vi "USRP SFP.vi"(0 "sfp 0.resources":T2, 5 "sfp 1.resources":T1) -> ()   [LabVIEW 2016]
uses:
  <instrlib>/_niInstr/CLIP Adapters/v1/FPGA/AXI4-Stream/Writer FXP64x1/niInstr AXI4-Stream Writer FXP64x1 v1 FPGA.lvclass
  <instrlib>/_niInstr/CLIP Adapters/v1/FPGA/AXI4-Stream/Reader FXP64x1/niInstr AXI4-Stream Reader FXP64x1 v1 FPGA.lvclass
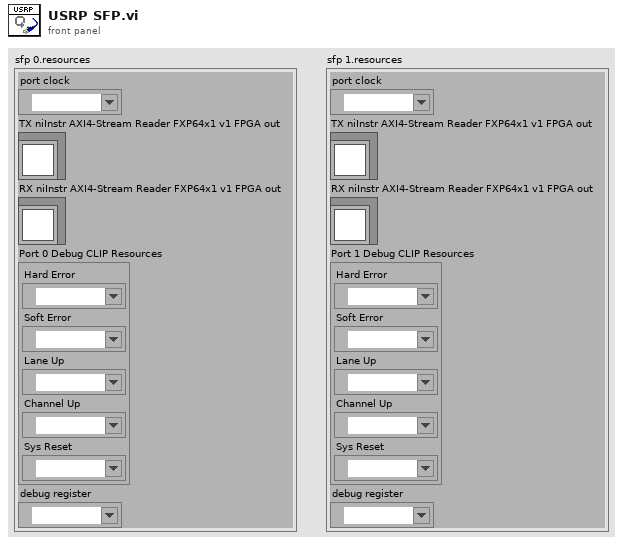
[diagram p1: front panel]
types:
  T1 = cluster{"port clock":refnum<k21>, "TX niInstr AXI4-Stream Reader FXP64x1 v1 FPGA out":refnum<class "niInstr AXI4-Stream Writer FXP64x1 v1 FPGA.lvclass">, "RX niInstr AXI4-Stream Reader FXP64x1 v1 FPGA out":refnum<class "niInstr AXI4-Stream Reader FXP64x1 v1 FPGA.lvclass">, "Port 1 Debug CLIP Resources":cluster{"Hard Error":refnum<k21>, "Soft Error":refnum<k21>, "Lane Up":refnum<k21>, "Channel Up":refnum<k21>, "Sys Reset":refnum<k21>}, "debug register":refnum<k21>}
  T2 = cluster{"port clock":refnum<k21>, "TX niInstr AXI4-Stream Reader FXP64x1 v1 FPGA out":refnum<class "niInstr AXI4-Stream Writer FXP64x1 v1 FPGA.lvclass">, "RX niInstr AXI4-Stream Reader FXP64x1 v1 FPGA out":refnum<class "niInstr AXI4-Stream Reader FXP64x1 v1 FPGA.lvclass">, "Port 0 Debug CLIP Resources":cluster{"Hard Error":refnum<k21>, "Soft Error":refnum<k21>, "Lane Up":refnum<k21>, "Channel Up":refnum<k21>, "Sys Reset":refnum<k21>}, "debug register":refnum<k21>}
  T3 = cluster{"Hard Error":refnum<k21>, "Soft Error":refnum<k21>, "Lane Up":refnum<k21>, "Channel Up":refnum<k21>, "Sys Reset":refnum<k21>}
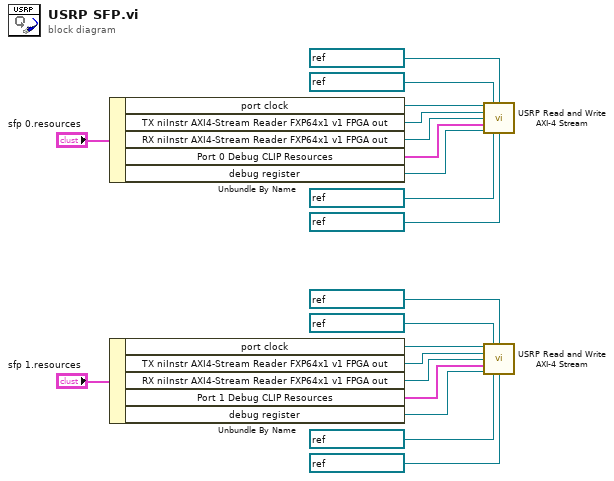
[diagram p0: block diagram]
diagram:
  n1 = Unbundle By Name("sfp 0.resources") -> ("port clock"=w11:refnum<k21>, "TX niInstr AXI4-Stream Reader FXP64x1 v1 FPGA out"=w10:refnum<class "niInstr AXI4-Stream Writer FXP64x1 v1 FPGA.lvclass">, "RX niInstr AXI4-Stream Reader FXP64x1 v1 FPGA out"=w9:refnum<class "niInstr AXI4-Stream Reader FXP64x1 v1 FPGA.lvclass">, "Port 0 Debug CLIP Resources"=w8:T3, "debug register"=w7:refnum<k21>)
  n2 = Unbundle By Name("sfp 1.resources") -> ("port clock"=w5:refnum<k21>, "TX niInstr AXI4-Stream Reader FXP64x1 v1 FPGA out"=w3:refnum<class "niInstr AXI4-Stream Writer FXP64x1 v1 FPGA.lvclass">, "RX niInstr AXI4-Stream Reader FXP64x1 v1 FPGA out"=w4:refnum<class "niInstr AXI4-Stream Reader FXP64x1 v1 FPGA.lvclass">, "Port 1 Debug CLIP Resources"=w2:T3, "debug register"=w1:refnum<k21>)
  n3 = call "USRP Read and Write AXI-4 Stream.vi"("port clock"=w11, "rx 0.sfp fifo"=refnum<k21> "rx 0.sfp 0 fifo" ("FIFO"), "rx 1.sfp fifo"=refnum<k21> "rx 1.sfp 0 fifo" ("FIFO"), "TX niInstr AXI4-Stream Reader FXP64x1 v1 FPGA out"=w10, "RX niInstr AXI4-Stream Reader FXP64x1 v1 FPGA out"=w9, "port debug CLIP resources"=w8, "port debug info"=w7, "tx 0.sfp fifo"=refnum<k21> "tx 0.sfp 0 fifo" ("FIFO"), "tx 1.sfp fifo"=refnum<k21> "tx 1.sfp 0 fifo" ("FIFO")) -> ()  [unwired: 7 in]
  n4 = call "USRP Read and Write AXI-4 Stream.vi"("port clock"=w5, "rx 0.sfp fifo"=refnum<k21> "rx 0.sfp 1 fifo" ("FIFO"), "rx 1.sfp fifo"=refnum<k21> "rx 1.sfp 1 fifo" ("FIFO"), "TX niInstr AXI4-Stream Reader FXP64x1 v1 FPGA out"=w3, "RX niInstr AXI4-Stream Reader FXP64x1 v1 FPGA out"=w4, "port debug CLIP resources"=w2, "port debug info"=w1, "tx 0.sfp fifo"=refnum<k21> "tx 0.sfp 1 fifo" ("FIFO"), "tx 1.sfp fifo"=refnum<k21> "tx 1.sfp 1 fifo" ("FIFO")) -> ()  [unwired: 7 in]
